vi "Initialize.vi"(8 "error in":errorcluster, 10 "parameters":variant, 11 "node in":refnum<class "Page.lvclass">) -> (0 "error out":errorcluster, 2 "summary":T2[](array[typedef]), 3 "data value reference":T1)   [LabVIEW 2015, in "Page.lvclass"]
doc: "Initializes the data of a node to its default state.\nThe object is not created inside of this VI, because it is created from a File depending on user selection."
uses:
  Page.lvclass
  <vilib>/NI/Configuration Framework/Node/Summary.ctl
  <vilib>/NI/Configuration Framework/Node/NodeRef.ctl
  <vilib>/NI/Configuration Framework/Node/NISE_CEF_Node.lvclass
  Page.lvclass/Page.ctl
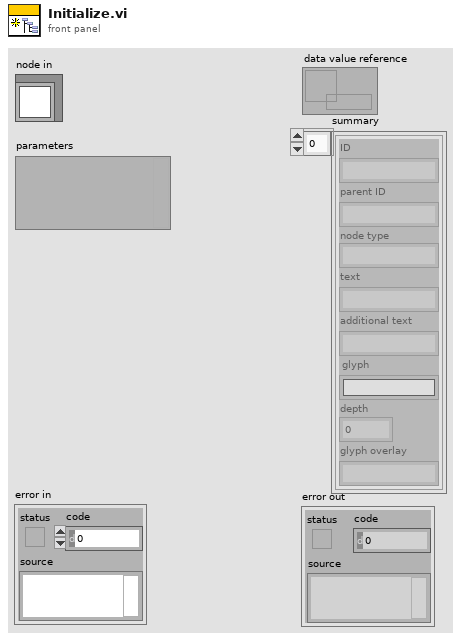
[diagram p1: front panel]
types:
  T1 = typedef "NISE_CEF_Node.lvclass/NodeRef.ctl" = refnum<data-value>
  T2 = typedef "NISE_CEF_Node.lvclass/Summary.ctl" = cluster{"ID":string, "parent ID":string, "node type":string, "text":string, "additional text":string, "glyph":string, "depth":i32, "glyph overlay":string}
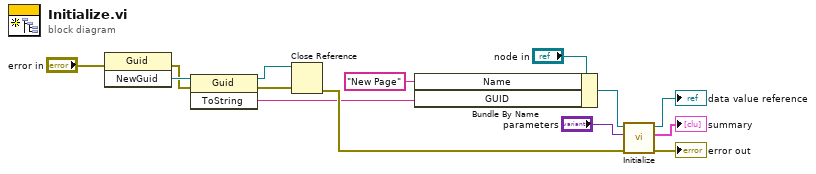
[diagram p0: block diagram]
diagram:
  n1 = invoke class="Guid" method="NewGuid"(error in="error in") -> (error out=w4:errorcluster, "NewGuid"=w6:refnum<k24>)  [unwired: 2 in, 1 out]
  n2 = invoke class="Guid" method="ToString"(reference=w6, error in=w4) -> (reference out=w7:refnum<k24>, error out=w3:errorcluster, "ToString"=w1:string)  [unwired: 1 in]
  n3 = Close Reference(reference=w7, error in (no error)=w3) -> (error out=w2:errorcluster)
  n4 = Bundle By Name(cluster="node in", "Name"="New Page" ("General Page Properties.Name"), "GUID"=w1) -> (w9:refnum<class "Page.lvclass">)
  n5 = call-parent "Initialize.vi"("error in"=w2, "parameters"="parameters", "node in"=w9) -> ("error out"=→"error out":errorcluster, "summary"=→"summary":T2[], "data value reference"=→"data value reference":T1)  [unwired: 6 in]
